vi "Read Status Calculation.vi"(8 "error in (no error)":errorcluster, 11 "abs_Parallel in":refnum<class "bt_Parallel.lvclass">) -> (0 "error out":errorcluster, 2 "Status Calculation":T1, 3 "abs_Parallel out":refnum<class "bt_Parallel.lvclass">)   [LabVIEW 2021, in "BT.lvlib" / "bt_Parallel.lvclass"]
uses:
  bt_Parallel.lvclass
  bt_Parallel.lvclass/bt_Parallel.ctl
  Support/Status Calculation.ctl
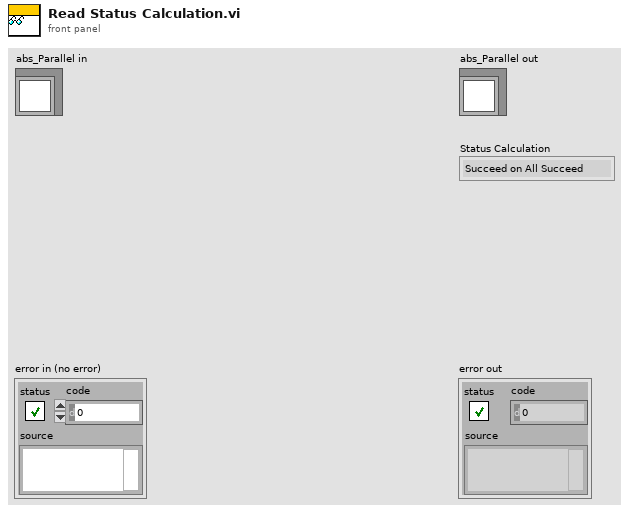
[diagram p1: front panel]
types:
  T1 = typedef "BT.lvlib/bt_Parallel.lvclass/Status Calculation.ctl" = enum16{"Succeed on All Succeed", "Failure on All Failure", "Succeed on Any Succeed", "Failure on Any Failure"}
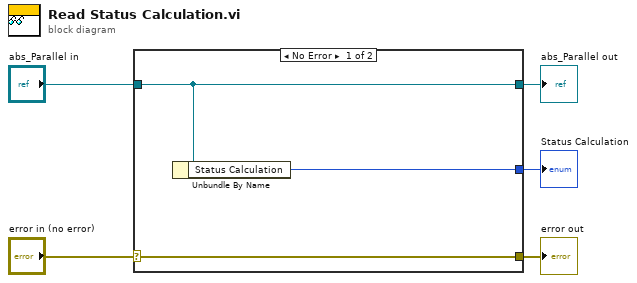
[diagram p0: block diagram]
diagram:
  n1 = case shown="No Error" "error in (no error)" {
    selector: "error in (no error)" -> [w8 w9]
    tunnel: [w8 w9] -> w4
    tunnel: [w7 w10] -> w2
    tunnel: "abs_Parallel in" -> [w7 w10]
    tunnel: [w6 _] -> w1
    frame No Error {
      n2 = Unbundle By Name(w7) -> ("Status Calculation"=w6:T1)
    }
    frame Error {
    }
  }
  "error out" <- w4
  "abs_Parallel out" <- w2
  "Status Calculation" <- w1
